vi "Free Label Color Applicator.vi"(10 "Dark Text?":bool=TRUE, 11 "Text Labels":refnum<vi>[](array[refnum])) -> ()   [LabVIEW 2021]
doc: "helper VI to color the free labels on the views that are plugged into the material theme editor\n\n<b>Code Developed By:</b> +\nDaniel Coons +\nTechnology Service Corporation +\nwww.tsc.com/atcs"
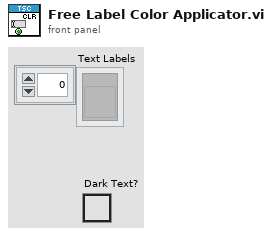
[diagram p1: front panel]
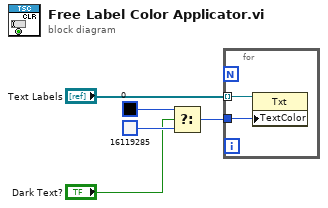
[diagram p0: block diagram]
diagram:
  n1 = Select(t=u32 0, s="Dark Text?", f=u32 16119285) -> (s? t:f=w1:u32)
  n2 = for {
    tunnel: "Text Labels" -> [w7] mode=indexing
    tunnel: w1 -> [w6]
    n3 = property on="Property Node" class="Txt"(reference=w7, "TextColor"=w6) -> ()  [unwired: 1 in, 2 out]
  }
